vi "2100_Test_Set State_Measure Resistance_SH3T_Rfree.vi"(0 "Semiconductor Module Context":T7, 1 "USID":T4 max=15, 2 "Publishable IDs":string[](array[string])=["State00", "State01", "State02", "State04", "State08"], 3 "R_Guardian":dbl[](array[numeric]), 5 "Script_Info":T3={"Script Name"="WalkingState", "All_Scripts"=[]}, 7 "Current  Level":dbl=0.01, 9 "Instrument_Pins":T6={"SMU_Pins"=["RF1", "RF2", "RF3", "RF4"], "HSDIO_Pins"=["CLK", "SDA"]}, 11 "Error In":errorcluster, 12 "Master_Register_Data_Array_In":T1 {"Address" format="%.0x"}, 13 "Reg_Map_and_Bit_Name":T5={"Reg_Map_Bit_Name"="", "Reg_Map"=[["Reg Addr(0x00)", "7", "6", "5", "4", "3", "2", "1", "0"], ["0", "SPARE", "RF3_SH", "RF2_SH", "RF1_SH", "SPARE", "RF3_RFC", "RF2_RFC", "RF1_RFC"], ["1", "SPARE[7:0]", "", "", "", "", "", "", ""], ["2", "VVAR_EN", "LCM_EN", "RFC_SH", "SPARE", "VARACTOR[3:0]", "", "", ""], ["3", "SW_CTRL1_VIRTUAL[7:0]", "", "", "", "", "", "", ""], ["4", "SW_CTRL1_SWAP", "SW_CTRL1_RBSHIFT[2:0]", "", "", "SW_CTRL1_VSID[3:0]", "", "", ""], ["5", "REG_00_VIRTUAL_MASK[7:0]", "", "", "", "", "", "", ""], ["6", "LOCK_STATUS[1:0]", "", "CLK_DITHER", "FUSES_BURNED", "CLK_IDAC_CAL[3:0]", "", "", ""], ["7", "SPARE[2:0]", "", "", "ODFT_TRIM[4:0]", "", "", "", ""], ["8", "SPARE[2:0]", "", "", "HV_TRIM[4:0]", "", "", "", ""], ["9", "TEST_MUX[2:0]", "", "", "SPARE[1:0]", "", "MEMS_BG_TC[1:0]", "", "MEMSCP_RCM"], ["A", "CP_BOOST_OVRD_EN", "SPARE[2:0]", "", "", "PS_OFF_TIMER[1:0]", "", "PS_ON_TIMER[1:0]", ""], ["0", "", "", "", "", "", "", "", ""], ["D", "Reserved[1:0]", "", "WD_HI_EVENT_CNT[5:0]", "", "", "", "", ""], ["E", "VERSION_ID[7:0]", "", "", "", "", "", "", ""], ["F", "Reserved", "COUNT_200_LSB[6:0]", "", "", "", "", "", ""], ["10", "CLK_DIV2_EN", "Spare", "ODFT_EN", "HV_HYST[4:0]", "", "", "", ""], ["0", "", "", "", "", "", "", "", ""], ["12", "SHORT_FUSE", "FUSE_BURN", "STROBE_EN", "VIO_OK", "RTH[1:0]", "", "FUSE_LOAD_MAN_EN", "FUSE_LOAD"], ["13", "RR_ACK_EN", "Reserved", "ACK_POSITION[1:0]", "", "SuBUS_DRIVE_STRENGTH[3:0]", "", "", ""], ["14", "TM_IO_EN", "TM_IO_SEL", "SuBUS_OVS[1:0]", "", "Reserved[3:0]", "", "", ""], ["15", "Reserved[4:0]", "", "", "", "", "SuBUS_VERSION_PRESENT", "SuBUS_VOLTAGE", "SuBUS_FLAVOR_DEF"], ["16", "PROG_STROBE1_DUR[7:0]", "", "", "", "", "", "", ""], ["17", "PROG_STROBE0_DUR[7:0]", "", "", "", "", "", "", ""], ["18", "Reserved[2:0]", "", "", "EFUSE_SINGLE_ADDR_SEL[4:0]", "", "", "", ""], ["19", "POLL_ADR[4:0]", "", "", "", "", "POLL_BC[2:0]", "", ""], ["1A", "SOFTWARE_RESET", "Reserved[6:0]", "", "", "", "", "", ""], ["1B", "Reserved[7:0]", "", "", "", "", "", "", ""], ["1C", "PWR_MODE_1", "PWR_MODE_0", "TRIGGER_MASK[2:0]", "", "", "TRIGGER[2:0]", "", ""], ["1D", "PRODUCT_ID[7:0]", "", "", "", "", "", "", ""], ["1E", "MANUFACTURER_ID_LSB[7:0]", "", "", "", "", "", "", ""], ["1F", "MANUFACTURER_ID_MSB[3:0]", "", "", "", "USID[3:0]", "", "", ""]]}) -> (6 "Master_Register_Data_Array_Out":T1 {"Address" format="%.0x"}, 15 "Error Out":errorcluster)   [LabVIEW 2013]
uses:
  Controls/USID.ctl
  <vilib>/NI_TestStand_SemiconductorModule/NI_TestStand_Semiconductor_Module.lvlibp/PinMap/General/SemiconductorModuleContext.ctl
  Controls/Master_Reg_Data_Array.ctl
  Controls/Reg_Address_Data.ctl
  <vilib>/NI_TestStand_SemiconductorModule/NI_TestStand_Semiconductor_Module.lvlibp/PinMap/General/Publish/PublishDataDoubleFunctionalTest.vi
  <vilib>/NI_TestStand_SemiconductorModule/NI_TestStand_Semiconductor_Module.lvlibp
panel:
  out "Data_Names":string[](array[string])
  out "Logged_Data":dbl[](array[numeric]) format="%#_6p"
  out "R_Measurements":dbl[][](array[numeric]) format="%#_6p"
  in  "Tab Control":enum32{"Test Info", "Instrument Settings"}(tab)
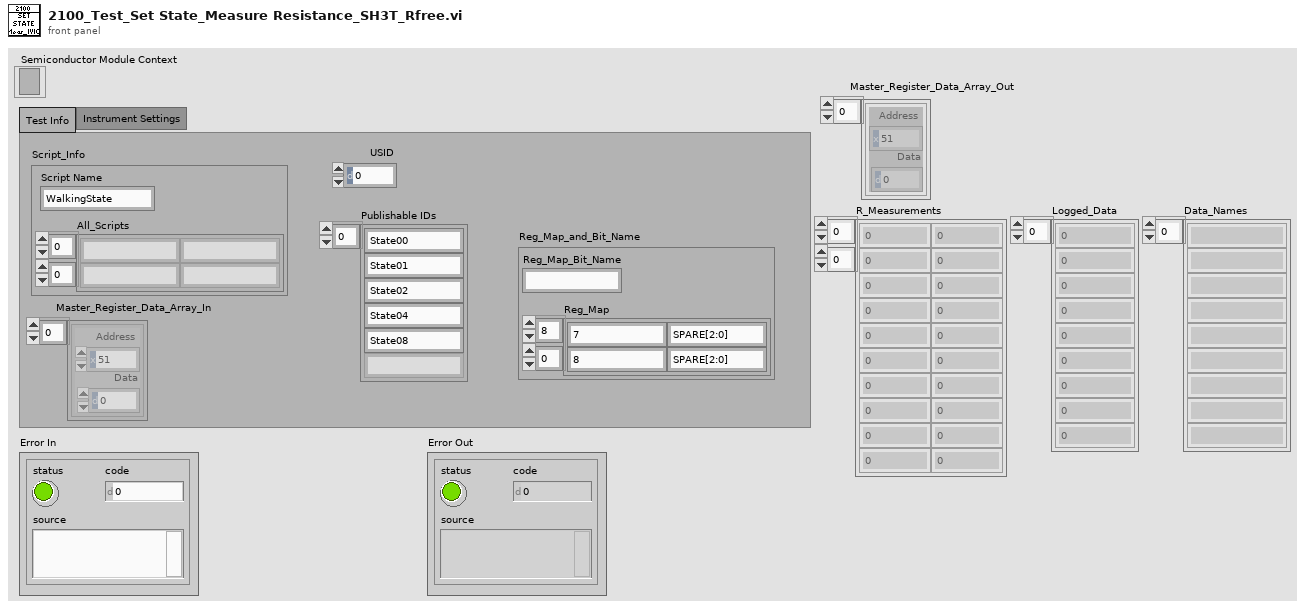
[diagram p1: front panel]
types:
  T1 = typedef "Master_Reg_Data_Array.ctl" = T2[]
  T2 = typedef "Reg_Address_Data.ctl" = cluster{"Address":u8, "Data":u8}
  T3 = cluster{"Script Name":string, "All_Scripts":string[][]}
  T4 = typedef "USID.ctl" = u8
  T5 = cluster{"Reg_Map_Bit_Name":string, "Reg_Map":string[][]}
  T6 = cluster{"SMU_Pins":string[], "HSDIO_Pins":string[]}
  T7 = typedef "NI_TestStand_Semiconductor_Module.lvlibp/SemiconductorModuleContext.ctl" = refnum<k7>
  T8 = typedef "Script Functions_Array.ctl" = enum16{"Reg_Write", "Bit_Write", "Delay", "Read", "Measure"}[]
  T9 = enum16{"Reg_Write", "Bit_Write", "Delay", "Read", "Measure"}
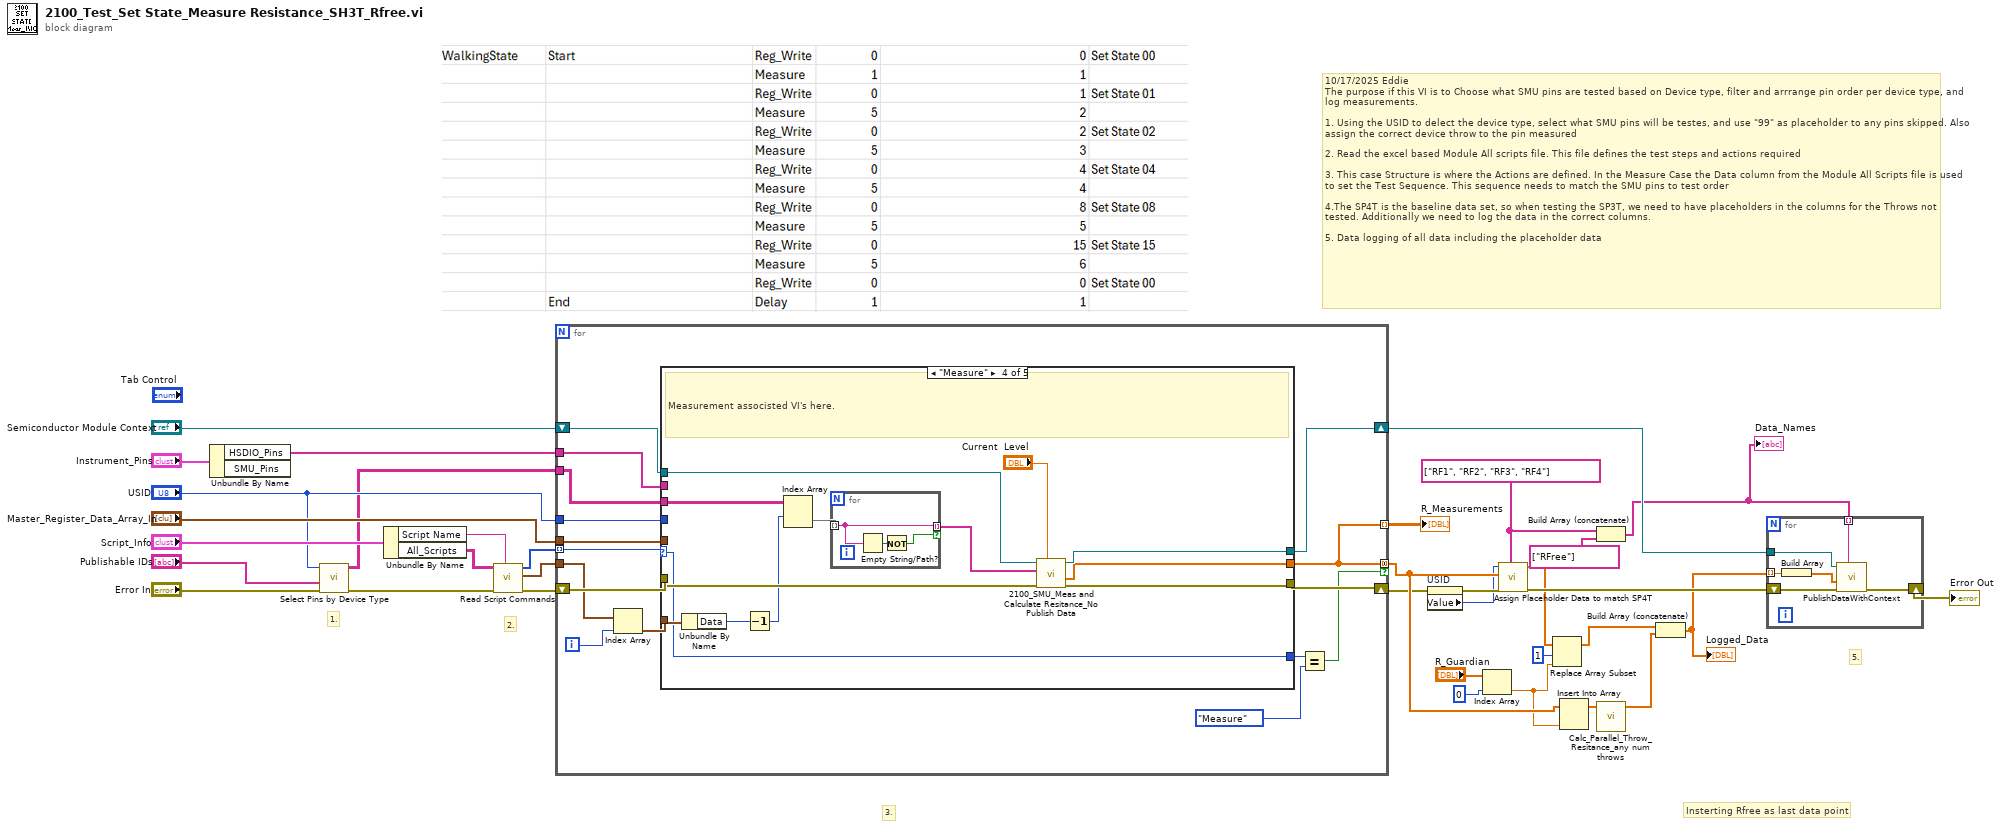
[diagram p0: block diagram]
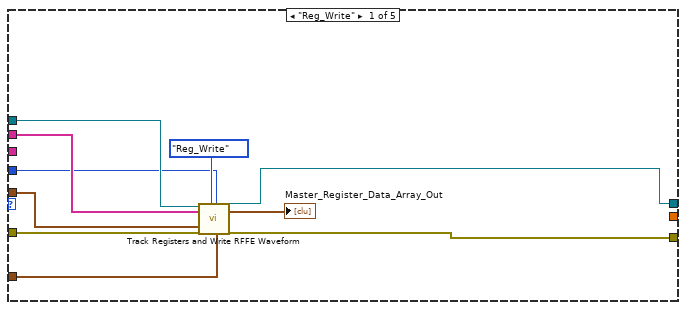
[diagram p2: hidden frame]
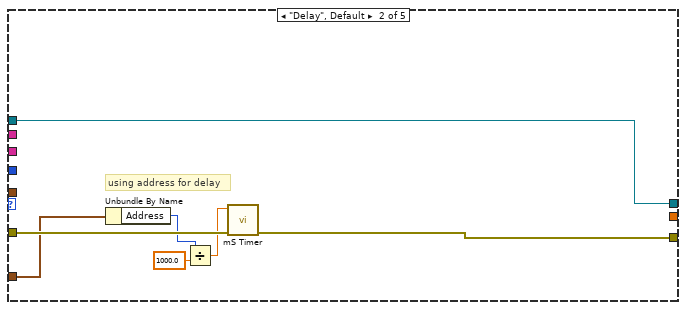
[diagram p3: hidden frame]
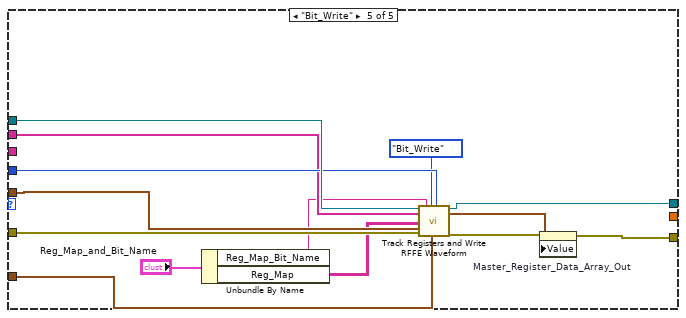
[diagram p5: hidden frame]
diagram:
  w16 = string[] ["RF1", "RF2", "RF3", "RF4"] ("SP4T_Pins")
  # "Insterting Rfree as last data point"
  # "10/17/2025 Eddie \nThe purpose if this VI is to Choose what SMU pins are tested based on Device type, filter and arrrange pin order per device type, and log measurements.\n\n1. Using the USID to delect the device type, select what SMU pins will be testes, and use \"99\" as placeholder to any pins skipped. Also assign the correct device throw to the pin measured\n\n2. Read the excel based Module All scripts file. This file defines the test steps and actions required\n\n3. This case Structure is where the Actions are defined. In the Measure Case the Data column from the Module All Scripts file is used to set the Test Sequence. This sequence needs to match the SMU pins to test order\n\n4.The SP4T is the baseline data set, so when testing the SP3T, we need to have placeholders in the columns for the Throws not tested. Additionally we need to log the data in the correct columns.\n\n5. Data logging of all data including the placeholder data"
  # "5."
  # "3."
  # "2."
  # "1."
  n1 = Unbundle By Name("Instrument_Pins") -> ("HSDIO_Pins"=w28:string[])  [unwired: 1 out]
  n2 = call "Select Pins by Device Type.vi"("error in (no error)"="Error In", "Publishable IDs"="Publishable IDs", "USID"="USID") -> ("error out"=w23:errorcluster, "Pins to Test"=w21:string[][])  [unwired: 7 in]
  n3 = Unbundle By Name("Script_Info") -> ("Script Name"=w25:string, "All_Scripts"=w26:string[][])
  n4 = call "Read Script Commands.vi"("Test Name"=w25, "Error In"=w23, "All_Scripts"=w26) -> ("Error Out"=w33:errorcluster, "Script_Data"=w34:T2[], "Script_Functions"=w35:T8)  [unwired: 5 in, 1 out]
  n5 = for {
    tunnel: "USID" -> [w45]
    tunnel: w35 -> [w44] mode=indexing
    tunnel: w34 -> [w48]
    tunnel: w28 -> [w49]
    shift-right: [w42] -> w3
    shift-left: w33 -> [w51]
    tunnel: "Master_Register_Data_Array_In" -> [w46]
    tunnel: [w40] -> w31 mode=indexing
    tunnel: w21 -> [w41]
    tunnel: [w40] -> w8 mode=concatenating if=w36
    shift-right: [w39] -> w19
    shift-left: "Semiconductor Module Context" -> [w50]
    i -> [w43]
    n6 = Index Array(array=w48, index=w43) -> (element=w47:T2)
    n7 = case shown="\"Measure\"" w44 {
      selector: w44 -> [_ _ _ w72 _]
      tunnel: w47 -> [w56 w67 _ w79 w87]
      tunnel: w51 -> [w61 w68 w70 w82 w100]
      tunnel: w45 -> [w53 _ _ _ w94]
      tunnel: w50 -> [w59 w62 w69 w81 w95]
      tunnel: w49 -> [w58 _ _ _ w92]
      tunnel: [w60 w66 w70 w83 w98] -> w42
      tunnel: w46 -> [w55 _ _ _ w91]
      tunnel: [_ _ _ w73 _] -> w40
      tunnel: w41 -> [_ _ _ w78 _]
      tunnel: [w52 w62 w69 w77 w96] -> w39
      tunnel: [_ _ _ w72 _] -> w38
      frame "Reg_Write" {
        n8 = call "Track Registers and Write RFFE Waveform.vi"("Semiconductor Module Context"=w59, "Pins"=w58, "Master_Register_Data_Array_In"=w55, "Error In"=w61, "Script_Functions"=enum16{"Reg_Write", "Bit_Write"}."Reg_Write", "USID"=w53, "Reg_Address_Data"=w56) -> ("Semiconductor Module Context Out"=w52:T7, "Master_Register_Data_Array_Out"=→"Master_Register_Data_Array_Out":T1, "Error Out"=w60:errorcluster)  [unwired: 10 in]
      }
      frame "Delay", Default {
        # "using address for delay"
        n9 = Unbundle By Name(w67) -> ("Address"=w64:u8)
        n10 = Divide(x=w64, y=1000.0) -> (x/y=w63:dbl)
        n11 = call "mS Timer.vi"("Error In"=w68, "Delay(S)"=w63) -> ("Error Out"=w66:errorcluster)  [unwired: 9 in]
      }
      frame "Read" {
        # "Future Dev Code"
      }
      frame "Measure" {
        # "Measurement associsted VI's here."
        n12 = Unbundle By Name(w79) -> ("Data"=w75:u8)
        n13 = Decrement(x=w75) -> (x-1=w74:u8)
        n14 = Index Array(array=w78, index (row)=w74) -> (element=w76:string[])  [unwired: 1 in]
        n15 = for {
          tunnel: w76 -> [w86] mode=indexing
          tunnel: [w86] -> w71 mode=indexing if=w84
          n16 = Empty String/Path?(string/path=w86) -> (empty?=w85:bool)
          n17 = Not(x=w85) -> (.not. x?=w84:bool)
        }
        n18 = call "2100_SMU_Meas and Calculate Resitance_No Publish Data.vi"("Current  Level"="Current  Level", "error in (no error)"=w82, "Pins"=w71, "Semiconductor Module Context"=w81) -> ("error Out"=w83:errorcluster, "Individual_R_Meas"=w73:dbl[], "Semiconductor Module Context Out"=w77:T7)  [unwired: 5 in]
      }
      frame "Bit_Write" {
        n19 = Unbundle By Name("Reg_Map_and_Bit_Name") -> ("Reg_Map_Bit_Name"=w89:string, "Reg_Map"=w88:string[][])
        n20 = call "Track Registers and Write RFFE Waveform.vi"("Semiconductor Module Context"=w95, "Pins"=w92, "Reg_Map"=w88, "Master_Register_Data_Array_In"=w91, "Error In"=w100, "Reg_Map_Bit_Name"=w89, "Script_Functions"=enum16{"Reg_Write", "Bit_Write"}."Bit_Write", "USID"=w94, "Reg_Address_Data"=w87) -> ("Semiconductor Module Context Out"=w96:T7, "Master_Register_Data_Array_Out"=w97:T1, "Error Out"=w99:errorcluster)  [unwired: 8 in]
        n21 = property on="Master_Register_Data_Array_Out" class="Arr (strict)"(error in=w99, "Value"=w97) -> (error out=w98:errorcluster)  [unwired: 1 in, 1 out]
      }
    }
    n22 = Equal?(x=w38, y=T9."Measure" ("Enum")) -> (x = y?=w36:bool)
  }
  "R_Measurements" <- w31
  n23 = property on="USID" class="DigNum (strict)"(error in=w3) -> (error out=w2:errorcluster, "Value"=w1:T4)  [unwired: 1 in, 1 out]
  n24 = Index Array(array="R_Guardian", index=0) -> (element=w7:dbl)
  n25 = call "Assign Placeholder Data to match SP4T.vi"("SP4T_Pins"=w16, "error in (no error)"=w2, "Individual_R_Meas"=w8, "USID"=w1) -> ("error out"=w17:errorcluster, "Placeholder_w_Data"=w11:dbl[])  [unwired: 6 in]
  n26 = Replace Array Subset(array=w11, new element=w7, index=1) -> (w5:dbl[])
  n27 = Insert Into Array(array=w8, new element=w7) -> (w9:dbl[])  [unwired: 1 in]
  n28 = Build Array (concatenate)(w16, string[] ["RFree"] ("element")) -> (w14:string[])
  "Data_Names" <- w14
  n29 = call "Calc_Parallel_Throw_Resitance_any num throws.vi"("Resitance_Per Site"=w9) -> ("Parallel_Resitance"=w6:dbl[])  [unwired: 10 in]
  n30 = Build Array (concatenate)(w5, w6) -> (w4:dbl[])
  "Logged_Data" <- w4
  n31 = for {
    shift-right: [w106] -> w20
    shift-left: w17 -> [w105]
    tunnel: w19 -> [w104]
    tunnel: w14 -> [w103] mode=indexing
    tunnel: w4 -> [w102] mode=indexing
    n32 = Build Array(w102) -> (w101:dbl[])
    n33 = call-poly <vilib>:"PublishDataWithContext.vi"("Published Data Id"=w103, "error in (no error)"=w105, "Data In"=w101, "Semiconductor Module Context"=w104) -> ("error out"=w106:errorcluster)  [unwired: 6 in, 1 out]
  }
  "Error Out" <- w20
